vi "Resolve Config Relative Path.vi"(8 "error in (no error)":errorcluster, 10 "Path":path, 11 "VolatusAPI in":refnum<class "VolatusAPI.lvclass">) -> (0 "error out":errorcluster, 2 "Resolved Path":path, 3 "VolatusAPI out":refnum<class "VolatusAPI.lvclass">)   [LabVIEW 2020, in "Volatus.lvlib" / "VolatusAPI.lvclass"]
uses:
  VolatusAPI.lvclass
  VolatusAPI.lvclass/VolatusAPI.ctl
  Volatus.lvlib
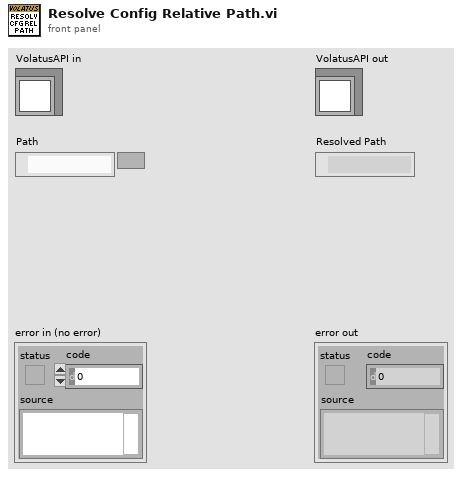
[diagram p1: front panel]
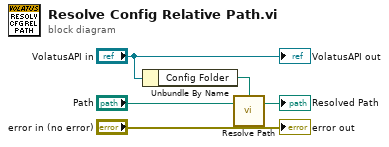
[diagram p0: block diagram]
diagram:
  n1 = Unbundle By Name("VolatusAPI in") -> ("Config Folder"=w3:path)
  n2 = call "Resolve Path.vi"("Starting Path"=w3, "Path"="Path") -> ("Resolved Path"=→"Resolved Path":path)  [unwired: 4 in]
  "error out" <- "error in (no error)"
  "VolatusAPI out" <- "VolatusAPI in"
